vi "HEXAA INTERVIEW QUESTION.vi"() -> ()   [LabVIEW 2020]
panel:
  in  "stop":bool
  out "Numeric 2":i32
  out "Numeric":i32
  in  "Boolean 2":bool
  in  "Boolean":bool
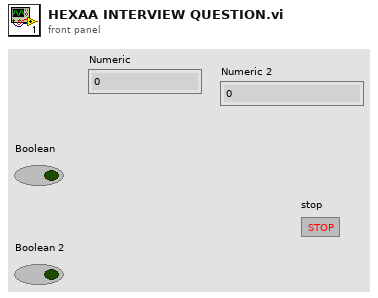
[diagram p1: front panel]
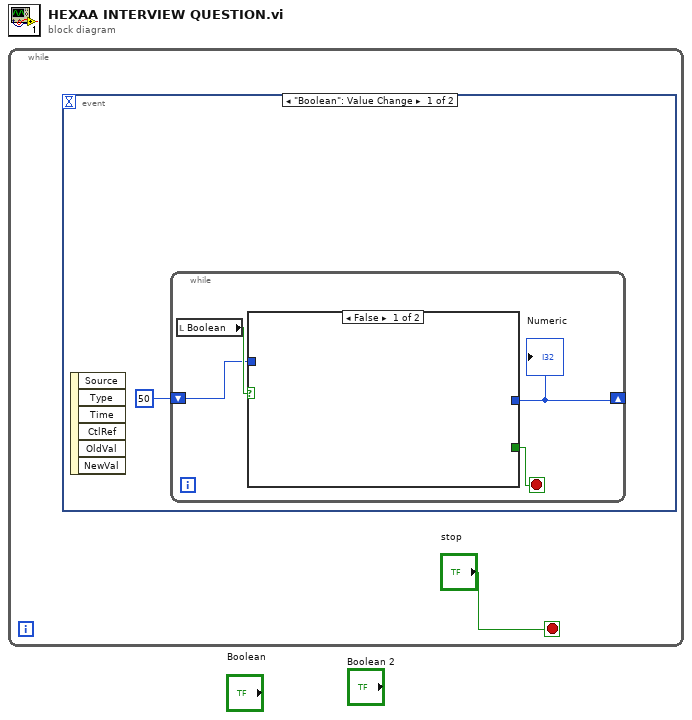
[diagram p0: block diagram]
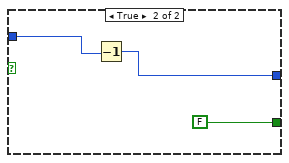
[diagram p2: hidden frame]
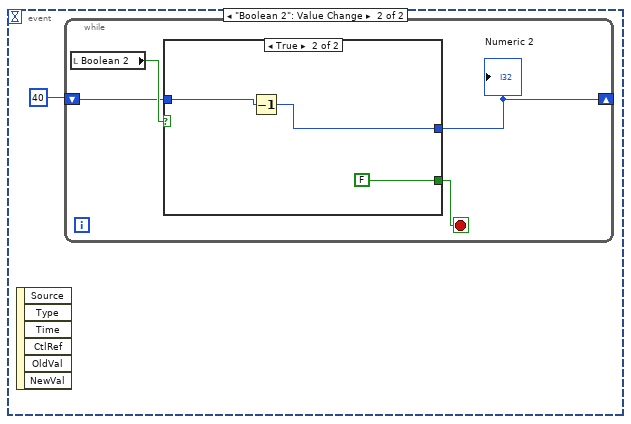
[diagram p3: hidden frame]
diagram:
  n1 = while {
    stop <- "stop" stop-if-true
    n2 = event shown="[0] \"Boolean\": Value Change" {
      selector: _ -> [_ _]
      dyn-events: _ -> [_ _]
      timeout: _ -> [_ _]
      event "Boolean": Value Change {
        n3 = event-data() -> ()  [unwired: 1 in, 6 out]
        n4 = while {
          shift-right: [w3] -> _
          shift-left: 50 -> [w5]
          stop <- w4 stop-if-true
          n5 = local read "Boolean"() -> (w6:bool)
          n6 = case shown="False" w6 {
            tunnel: w5 -> [_ w9]
            tunnel: [_ w8] -> w3
            tunnel: [_ FALSE] -> w4
            frame False {
            }
            frame True {
              n7 = Decrement(x=w9) -> (x-1=w8:i32)
            }
          }
          "Numeric" <- w3
        }
      }
      event "Boolean 2": Value Change {
        n8 = event-data() -> ()  [unwired: 1 in, 6 out]
        n9 = while {
          shift-right: [w11] -> _
          shift-left: 40 -> [w13]
          stop <- w12 stop-if-true
          n10 = local read "Boolean 2"() -> (w14:bool)
          n11 = case shown="True" w14 {
            tunnel: [_ w17] -> w11
            tunnel: w13 -> [_ w16]
            tunnel: [_ FALSE] -> w12
            frame False {
            }
            frame True {
              n12 = Decrement(x=w16) -> (x-1=w17:i32)
            }
          }
          "Numeric 2" <- w11
        }
      }
    }
  }
